vi "Test Attach Debugger to Uninitialized Process Throws Error.vi"(8 "error in (no error)":errorcluster, 11 "Test Case In":refnum<class "Attach Debugger.lvclass">) -> (0 "error out":errorcluster, 3 "Test Case Out":refnum<class "Attach Debugger.lvclass">)   [LabVIEW 2020, in "Attach Debugger.lvclass"]
uses:
  Attach Debugger.lvclass
  Attach Debugger.lvclass/Attach Debugger.ctl
  Test Process/Test Process.lvclass
  <vilib>/Astemes/LUnit/Test Case.lvclass
  C:/Program Files (x86)/National Instruments/LabVIEW 2020/vi.lib/Astemes/Triarc Framework/Process/Process.lvclass
  C:/Program Files (x86)/National Instruments/LabVIEW 2020/vi.lib/Astemes/LUnit/Test Case.lvclass
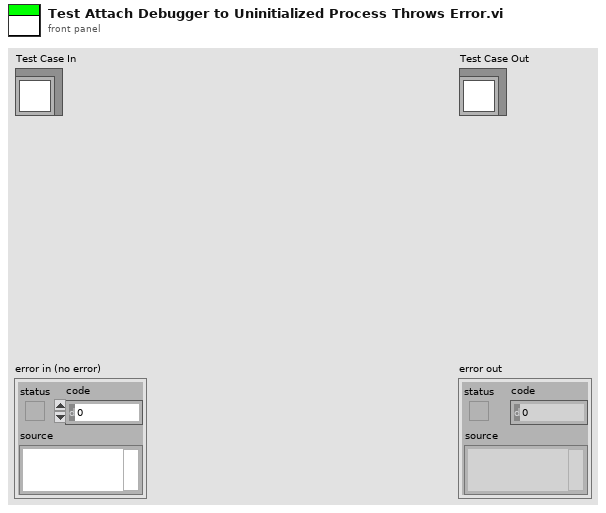
[diagram p1: front panel]
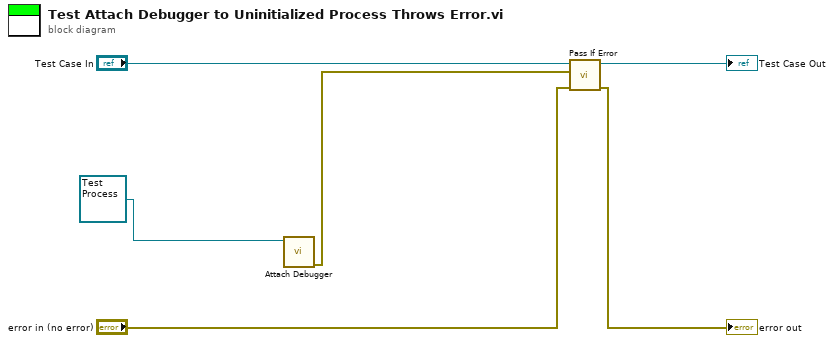
[diagram p0: block diagram]
diagram:
  n1 = call "Attach Debugger.vi"("Process In"=refnum<class "Test Process.lvclass"> refnum ("Test Process.lvclass")) -> ("error out"=w1:errorcluster)  [unwired: 10 in]
  n2 = call <vilib>:"Pass If Error.vi"("error in (no error)"="error in (no error)", "Assert error"=w1, "LUnit Test Case In"="Test Case In") -> ("error out"=→"error out":errorcluster, "LUnit Test Case Out"=→"Test Case Out":refnum<class "Attach Debugger.lvclass">)  [unwired: 7 in]
